vi "getNsamples.vi"(8 "error in (no error)":errorcluster, 11 "params":refnum<class "JSON Value.lvclass">) -> (0 "error out":errorcluster, 3 "data":refnum<class "JSON Value.lvclass">)   [LabVIEW 2017]
uses:
  <vilib>/NI/JSON Support for LabVIEW/JSON Value/JSON Value.lvclass
  <vilib>/DAQmx/read.llb/DAQmx Read (Analog 1D DBL 1Chan NSamp).vi
  <vilib>/NI/JSON Support for LabVIEW/JSON Value/Object/Get Value/Get Value (String).vi
  <vilib>/NI/JSON Support for LabVIEW/JSON Value/Object/Get Value/Get Value (Numeric).vi
  <vilib>/DAQmx/create/channels.llb/DAQmx Create Channel (AI-Voltage-Basic).vi
  <vilib>/DAQmx/configure/timing.llb/DAQmx Timing (Sample Clock).vi
  <vilib>/DAQmx/miscellaneous.llb/DAQmx Fill In Error Info.vi
  <vilib>/NI/JSON Support for LabVIEW/JSON Value/New JSON Value/New JSON (Numeric[]).vi
  <vilib>/NI/JSON Support for LabVIEW/JSON Value/New JSON Value/New JSON (Numeric).vi
  <vilib>/NI/JSON Support for LabVIEW/JSON Value/New JSON Value/New JSON ({Value[]}).vi
  <vilib>/NI/NI JSONRPC Server Framework/Classes/Server/JSONRPC Server.lvclass
  <resource>/objmgr/daqmx.rc
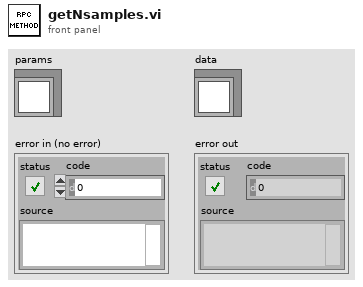
[diagram p1: front panel]
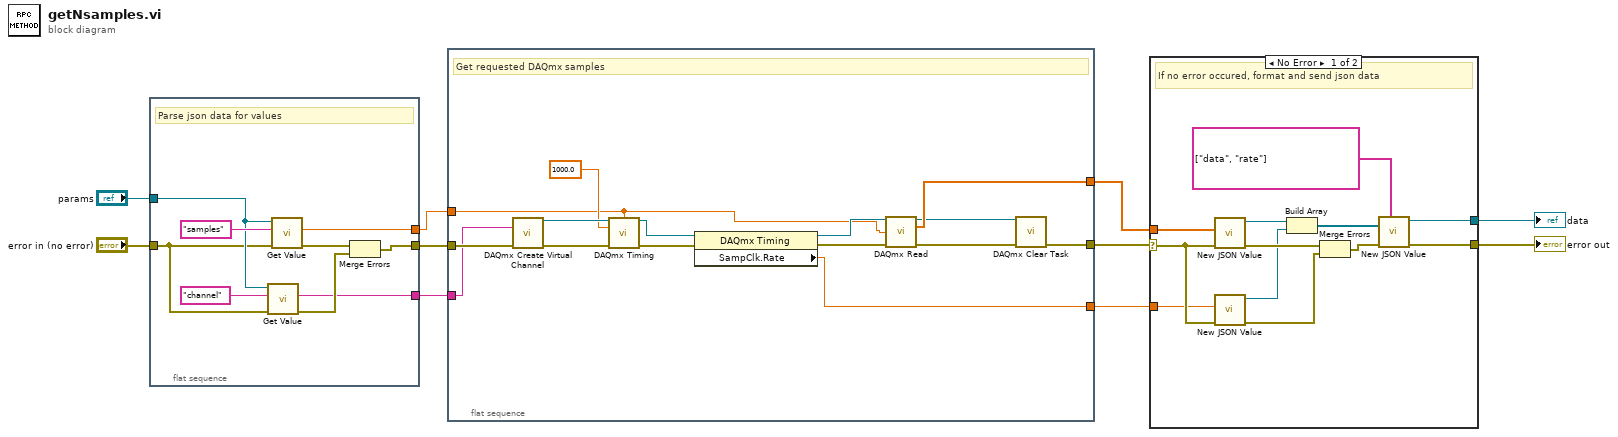
[diagram p0: block diagram]
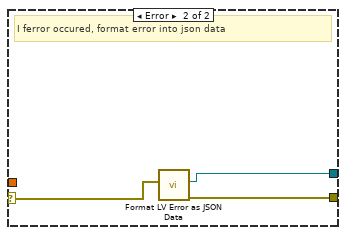
[diagram p2: hidden frame]
diagram:
  n1 = flat-sequence {
    tunnel: "params" -> [w17]
    tunnel: "error in (no error)" -> [w11]
    tunnel: [w15] -> w8
    tunnel: [w13] -> w2
    tunnel: [w12] -> w3
    frame #0 {
      # "Parse json data for values"
      n2 = call-poly <vilib>:"Get Value.vi"("error in (no error)"=w11, "key"="channel", "JSON Value in"=w17) -> ("error out"=w14:errorcluster, "value"=w12:string)  [unwired: 7 in]
      n3 = call-poly <vilib>:"Get Value.vi"("error in (no error)"=w11, "key"="samples", "JSON Value in"=w17) -> ("error out"=w16:errorcluster, "value"=w13:dbl)  [unwired: 7 in]
      n4 = Merge Errors(w16, w14) -> (w15:errorcluster)
    }
  }
  n5 = flat-sequence {
    tunnel: w8 -> [w34]
    tunnel: [w27] -> w5
    tunnel: [w23] -> w4
    tunnel: w3 -> [w33]
    tunnel: w2 -> [w24]
    tunnel: [w20] -> w1
    frame #0 {
      # "Get requested DAQmx samples"
      n6 = call-poly <vilib>:"DAQmx Create Virtual Channel.vi"("physical channels"=w33, "error in"=w34) -> ("task out"=w31:refnum<k21>, "error out"=w32:errorcluster)  [unwired: 12 in]
      n7 = call-poly <vilib>:"DAQmx Timing.vi"("task/channels in"=w31, "samples per channel"=w24, "rate"=1000.0, "error in"=w32) -> ("task out"=w28:refnum<k21>, "error out"=w29:errorcluster)  [unwired: 10 in]
      n8 = property class="DAQmx Timing"(reference=w28, error in=w29) -> (reference out=w25:refnum<k21>, error out=w26:errorcluster, "SampClk.Rate"=w27:dbl)
      n9 = call-poly <vilib>:"DAQmx Read.vi"("task/channels in"=w25, "number of samples per channel"=w24, "error in"=w26) -> ("task out"=w21:refnum<k21>, "data"=w23:dbl[], "error out"=w22:errorcluster)  [unwired: 10 in]
      n10 = call <vilib>:"DAQmx Clear Task.vi"("task in"=w21, "error in"=w22) -> ("error out"=w20:errorcluster)  [unwired: 13 in]
    }
  }
  n11 = case shown="No Error" w1 {
    selector: w1 -> [w40 w49]
    tunnel: [w45 w47] -> w7
    tunnel: [w39 w48] -> w6
    tunnel: w4 -> [w38 _]
    tunnel: w5 -> [w35 _]
    frame No Error {
      # "If no error occured, format and send json data"
      n12 = call-poly <vilib>:"New JSON Value.vi"("error in (no error)"=w40, "Numeric Array"=w38) -> ("error out"=w46:errorcluster, "JSON Value out"=w44:refnum<class "JSON Value.lvclass">)  [unwired: 8 in]
      n13 = call-poly <vilib>:"New JSON Value.vi"("error in (no error)"=w40, "value"=w35) -> ("error out"=w41:errorcluster, "JSON Value out"=w43:refnum<class "JSON Value.lvclass">)  [unwired: 8 in]
      n14 = Build Array(w44, w43) -> (w37:refnum<class "JSON Value.lvclass">[])
      n15 = Merge Errors(w46, w41) -> (w42:errorcluster)
      n16 = call-poly <vilib>:"New JSON Value.vi"("keys"=string[] ["data", "rate"], "error in (no error)"=w42, "values"=w37) -> ("error out"=w45:errorcluster, "JSON Value out"=w39:refnum<class "JSON Value.lvclass">)  [unwired: 7 in]
    }
    frame Error {
      # "I ferror occured, format error into json data"
      n17 = call <vilib>:"Format LV Error as JSON Data.vi"("error in"=w49) -> ("error out"=w47:errorcluster, "Error Value out"=w48:refnum<class "JSON Value.lvclass">)  [unwired: 9 in]
    }
  }
  "data" <- w6
  "error out" <- w7
